vi "Expand_control_ref_with_nested_controls.vi"(4 "error in (no error)":errorcluster, 7 "Control":refnum<vi>) -> (0 "error out":errorcluster, 3 "Array of control info":cluster{"Control":refnum<vi>, "Level":i32}[](array[cluster]))   [LabVIEW 2017, in "NI_ReportGenerationCore.lvlib"]
uses:
  <vilib>/Utility/NIReport.llb/NI_ReportGenerationCore.lvlib
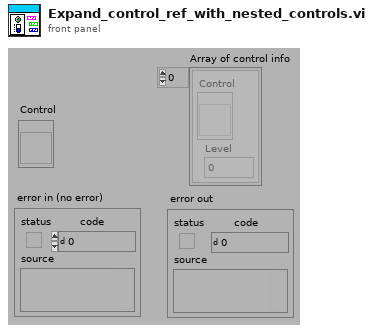
[diagram p1: front panel]
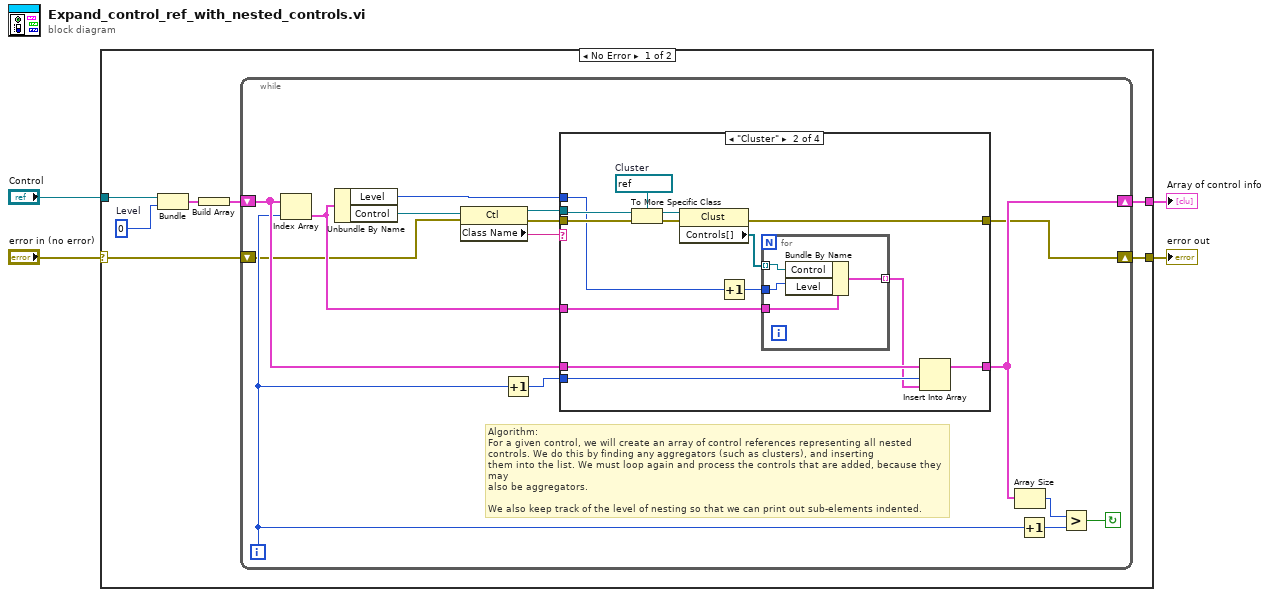
[diagram p0: block diagram]
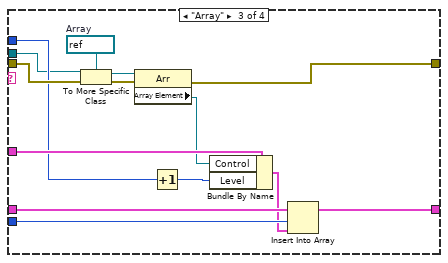
[diagram p3: hidden frame]
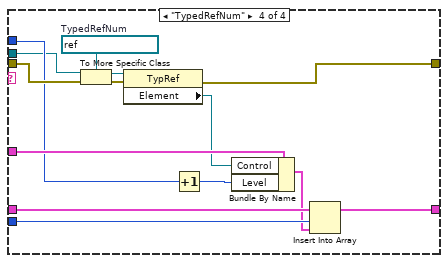
[diagram p4: hidden frame]
diagram:
  n1 = case shown="No Error" "error in (no error)" {
    selector: "error in (no error)" -> [w5 w75]
    tunnel: "Control" -> [w9 _]
    tunnel: [w7 _] -> w3
    tunnel: [w6 w75] -> w2
    frame No Error {
      w10 = 0  # Level
      n2 = Bundle("Control"=w9, "Level"=w10) -> (w8:cluster{"Control":refnum<vi>, "Level":i32})  [unwired: 1 in]
      n3 = Build Array(w8) -> (w11:cluster{"Control":refnum<vi>, "Level":i32}[])
      n4 = while {
        shift-right: [w18] -> w7
        shift-left: w11 -> [w23]
        shift-right: [w12] -> w6
        shift-left: w5 -> [w13]
        i -> [w22]
        stop <- w16 continue-if-true
        # "Algorithm:\nFor a given control, we will create an array of control references representing all nested\ncontrols. We do this by finding any aggregators (such as clusters), and inserting\nthem into the list. We must loop again and process the controls that are added, because they may\nalso be aggregators.\n\nWe also keep track of the level of nesting so that we can print out sub-elements indented."
        n5 = Index Array(array=w23, index=w22) -> (element=w19:cluster{"Control":refnum<vi>, "Level":i32})
        n6 = Unbundle By Name(w19) -> ("Level"=w20:i32, "Control"=w21:refnum<vi>)
        n7 = property class="Ctl"(reference=w21, error in=w13) -> (reference out=w26:refnum<vi>, error out=w24:errorcluster, "Class Name"=w25:string)
        n8 = Increment(x=w22) -> (x+1=w15:i32)
        n9 = case shown="\"Cluster\"" w25 {
          tunnel: w24 -> [w28 w41 w59 w73]
          tunnel: [w28 w38 w56 w70] -> w12
          tunnel: w26 -> [_ w37 w47 w61]
          tunnel: w23 -> [w27 w36 w55 w68]
          tunnel: w15 -> [_ w35 w54 w67]
          tunnel: [w27 w34 w53 w63] -> w18
          tunnel: w20 -> [_ w32 w50 w62]
          tunnel: w19 -> [_ w30 w52 w65]
          frame Default {
          }
          frame "Cluster" {
            w42 = refnum<vi> refnum  # Cluster
            n10 = To More Specific Class(target class=w42, reference=w37, error in=w41) -> (specific class reference=w40:refnum<vi>, error out=w39:errorcluster)
            n11 = property class="Clust"(reference=w40, error in=w39) -> (error out=w38:errorcluster, "Controls[]"=w33:refnum<vi>[])  [unwired: 1 out]
            n12 = Increment(x=w32) -> (x+1=w31:i32)
            n13 = for {
              tunnel: w33 -> [w45] mode=indexing
              tunnel: w31 -> [w44]
              tunnel: w30 -> [w46]
              tunnel: [w43] -> w29 mode=indexing
              n14 = Bundle By Name(cluster=w46, "Control"=w45, "Level"=w44) -> (w43:cluster{"Control":refnum<vi>, "Level":i32})
            }
            n15 = Insert Into Array(array=w36, index=w35, new element=w29) -> (w34:cluster{"Control":refnum<vi>, "Level":i32}[])
          }
          frame "Array" {
            w60 = refnum<vi> refnum  # Array
            n16 = To More Specific Class(target class=w60, reference=w47, error in=w59) -> (specific class reference=w58:refnum<vi>, error out=w57:errorcluster)
            n17 = property class="Arr"(reference=w58, error in=w57) -> (error out=w56:errorcluster, "Array Element"=w51:refnum<vi>)  [unwired: 1 out]
            n18 = Increment(x=w50) -> (x+1=w49:i32)
            n19 = Bundle By Name(cluster=w52, "Control"=w51, "Level"=w49) -> (w48:cluster{"Control":refnum<vi>, "Level":i32})
            n20 = Insert Into Array(array=w55, index=w54, new element=w48) -> (w53:cluster{"Control":refnum<vi>, "Level":i32}[])
          }
          frame "TypedRefNum" {
            w74 = refnum<vi> refnum  # TypedRefNum
            n21 = To More Specific Class(target class=w74, reference=w61, error in=w73) -> (specific class reference=w72:refnum<vi>, error out=w71:errorcluster)
            n22 = property class="TypRef"(reference=w72, error in=w71) -> (error out=w70:errorcluster, "Element"=w64:refnum<vi>)  [unwired: 1 out]
            n23 = Increment(x=w62) -> (x+1=w69:i32)
            n24 = Bundle By Name(cluster=w65, "Control"=w64, "Level"=w69) -> (w66:cluster{"Control":refnum<vi>, "Level":i32})
            n25 = Insert Into Array(array=w68, index=w67, new element=w66) -> (w63:cluster{"Control":refnum<vi>, "Level":i32}[])
          }
        }
        n26 = Array Size(array=w18) -> (size(s)=w17:i32)
        n27 = Increment(x=w22) -> (x+1=w14:i32)
        n28 = Greater?(x=w17, y=w14) -> (0:w16:bool)
      }
    }
    frame Error {
    }
  }
  "error out" <- w2
  "Array of control info" <- w3
